vi "Get Sender.vi"(11 "Create Msg Strategy in":refnum<class "Create Msg Strategy.lvclass">) -> (2 "Sender":refnum<class "Sender.lvclass">)   [LabVIEW 2021, in "Create Msg Strategy.lvlib" / "Create Msg Strategy.lvclass"]
uses:
  Create Msg Strategy.lvclass
  Create Msg Strategy.lvclass/Create Msg Strategy.ctl
  jettl/Sender/Sender/Sender.lvclass
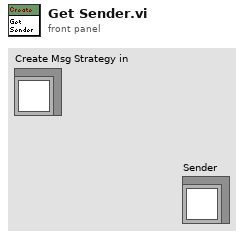
[diagram p1: front panel]
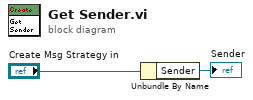
[diagram p0: block diagram]
diagram:
  n1 = Unbundle By Name("Create Msg Strategy in") -> ("Sender"=→"Sender":refnum<class "Sender.lvclass">)
